vi "Flame_ColorTemp_indicator_subVI.vi"(8 "pixel length":i32=1050, 9 "pixel index":i32=910, 11 "Color Temp":dbl[](array[numeric])) -> (0 "variance":dbl format="%0.2f", 2 "standard deviation":dbl format="%0.2f", 3 "Average Color temperature":dbl format="%0.2f")   [LabVIEW 2017]
uses:
  <vilib>/Analysis/NI_AALBase.lvlib
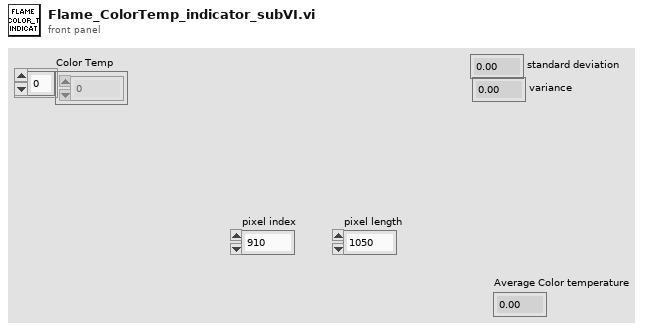
[diagram p1: front panel]
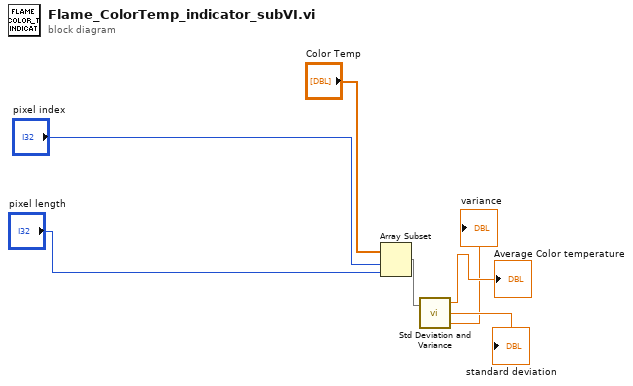
[diagram p0: block diagram]
diagram:
  n1 = Array Subset(array="Color Temp", index="pixel index", length="pixel length") -> (w4:dbl[])
  n2 = call <vilib>:"Std Deviation and Variance.vi"("X"=w4) -> ("mean"=→"Average Color temperature":dbl, "standard deviation"=→"standard deviation":dbl, "variance"=→"variance":dbl)  [unwired: 1 in]
